vi "AWS-Shared-MD5ofContent.vi"(5 "Content":string, 7 "Encoding":enum16{"base64", "ASCII Hex"}(ring), 11 "error in":errorcluster) -> (6 "MD5":string, 15 "error out":errorcluster)   [LabVIEW 2012]
uses:
  C:/Users/Jack/repo/visualize/Dependencies/aws/AWS-SDK/AWSSDK.dll
  AWS-SDK/AWSSDK.dll
panel:
  # "Inputs"
  # "Outputs"
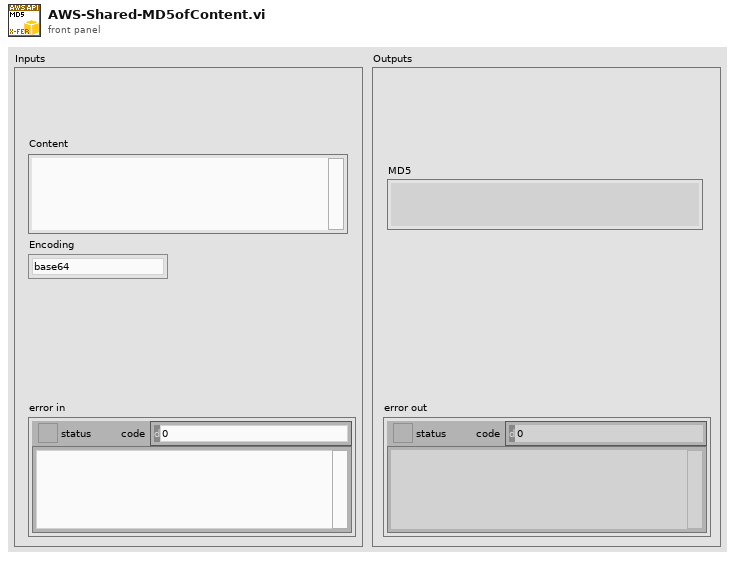
[diagram p1: front panel]
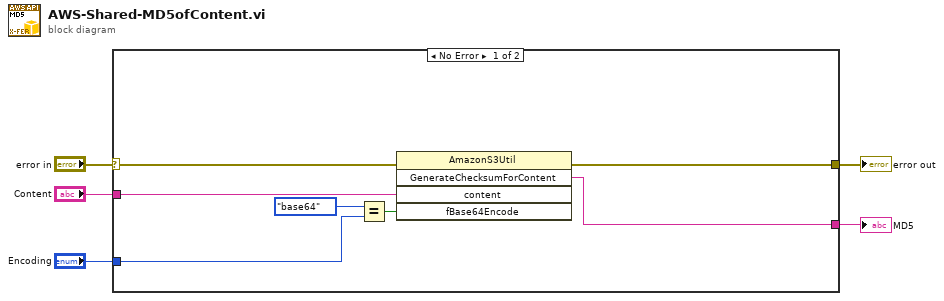
[diagram p0: block diagram]
diagram:
  n1 = case shown="No Error" "error in" {
    selector: "error in" -> [w6 w13]
    tunnel: [w8 w13] -> w5
    tunnel: [w12 _] -> w3
    tunnel: "Encoding" -> [w9 _]
    tunnel: "Content" -> [w7 _]
    frame No Error {
      n2 = Equal?(x=enum16{"base64", "ASCII Hex"}."base64" ("Encoding"), y=w9) -> (x = y?=w10:bool)
      n3 = invoke class="AmazonS3Util" method="GenerateChecksumForContent"(error in=w6, "content"=w7, "fBase64Encode"=w10) -> (error out=w8:errorcluster, "GenerateChecksumForContent"=w12:string)  [unwired: 2 in, 3 out]
    }
    frame Error {
    }
  }
  "error out" <- w5
  "MD5" <- w3
